vi "Continuous B sweep.vi"(6 "Mode":T2, 7 "Rate (T/min)":dbl=0.0125 min=0.0 max=0.2, 8 "error in (no error)":errorcluster, 9 "Simulate/Run":enum16{"simulate mode", "run mode"}(ring), 10 "Min (start)":dbl=1.0 min=-8.0 max=8.0, 11 "Max (end)":dbl=-1.0 min=-8.0 max=8.0) -> (0 "error out":errorcluster)   [LabVIEW 2019, in "Sweep Control.lvclass"]
uses:
  Sweep Control.lvclass
  Typedefs/Enum - Experiments.ctl
  Typedefs/Continuous B Sweep JSON--Cluster.ctl
  <userlib>/LevyLab/Transport/Transport/Transport.lvclass
  <userlib>/LevyLab/Transport/Control Experiment/Control Experiment.lvclass
  <userlib>/LevyLab/Instrument Framework/Instrument Types/Cryostat/Instrument.Cryostat.lvclass
  <userlib>/LevyLab/Transport/Control Experiment/Typedefs/Instrument Classes--cluster.ctl
  <userlib>/LevyLab/Transport/Control Experiment/Typedefs/Wiring Description--cluster.ctl
  <userlib>/LevyLab/Transport/Control Experiment/Typedefs/Experiment Description--cluster.ctl
  <userlib>/LevyLab/Instrument Framework/Instrument Types/VSource/Instrument.VSource.lvclass
  <userlib>/LevyLab/Instrument Framework/Instrument Types/VNA/Instrument.VNA.lvclass
  <userlib>/LevyLab/Instrument Framework/Instrument Types/Strain/Instrument.Strain.lvclass
  <userlib>/LevyLab/Instrument Framework/Instrument Types/CBridge/Instrument.CBridge.lvclass
  <userlib>/LevyLab/Lockin-Multichannel/Instrument.DAQ/Typedefs/Sweep.Pattern--Enum.ctl
  <userlib>/LevyLab/Lockin-Multichannel/Instrument.DAQ/Instrument.DAQ.lvclass
  <userlib>/LevyLab/Lockin-Multichannel/Instrument.DAQ/Typedefs/Sweep.Configuration--Cluster.ctl
  <userlib>/LevyLab/Instrument Framework/Instrument Types/Delay Line/Instrument.DelayLine.lvclass
  <userlib>/LevyLab/Lockin-Multichannel/Instrument.DAQ/Typedefs/REF.Channel--Cluster--Array.ctl
  <userlib>/LevyLab/Lockin-Multichannel/Instrument.DAQ/Typedefs/AO.Channel--Cluster--Array.ctl
  65c9b652-50f2-4ab4-8260-00ea008a43cc.vi
  <userlib>/LevyLab/Transport/Control Experiment/Typedefs/Instruments--cluster.ctl
  <userlib>/LevyLab/Krohn Hite 7008/KH7008/typedefs/Filter--Enum.ctl
  <userlib>/LevyLab/Krohn Hite 7008/KH7008/KH7008.lvlib
  <userlib>/LevyLab/Krohn Hite 7008/KH7008/typedefs/couple--Enum.ctl
  <userlib>/LevyLab/Krohn Hite 7008/KH7008/typedefs/shunt--enum.ctl
  <userlib>/LevyLab/Krohn Hite 7008/KH7008/typedefs/Input--Enum.ctl
  <userlib>/LevyLab/Krohn Hite 7008/KH7008/typedefs/gain--enum.ctl
  <userlib>/LevyLab/Krohn Hite 7008/KH7008/typedefs/channel--numeric.ctl
  <userlib>/LevyLab/Krohn Hite 7008/KH7008/typedefs/channelProperties--Cluster.ctl
  <userlib>/LevyLab/Krohn Hite 7008/KH7008/typedefs/allChannelProperties--Array.ctl
  <userlib>/LevyLab/Lockin-Multichannel/Instrument.DAQ/Typedefs/Sweep.Channel--Cluster.ctl
  <userlib>/LevyLab/Lockin-Multichannel/Instrument.DAQ/Typedefs/Sweep.Channel--Cluster--Array.ctl
  <userlib>/LevyLab/Instrument Framework/Instrument Types/Lockin/Instrument.LockinAPI.lvclass
  <userlib>/LevyLab/Instrument Framework/Instrument Types/Amplifier/Instrument.Amplifier.lvclass
  <userlib>/LevyLab/Lockin-Multichannel/Instrument.DAQ/Typedefs/AO.Channel.Function--Enum.ctl
  <userlib>/LevyLab/Lockin-Multichannel/Instrument.DAQ/Typedefs/AO.Channel--Cluster.ctl
  <userlib>/LevyLab/Lockin-Multichannel/Instrument.DAQ/Typedefs/REF.Channel--Cluster.ctl
  <userlib>/LevyLab/Lockin-Multichannel/Instrument.Lockin/Instrument.Lockin.lvclass
  <userlib>/LevyLab/Krohn Hite 7008/Inst.Krohn-Hite-7008/Inst.Krohn-Hite-7008.lvclass
  <userlib>/LevyLab/Instrument Framework/Instrument Types/Cryostat/Typedefs/Magnet Axis--Enum.ctl
  <userlib>/LevyLab/Transport/Control Experiment/Typedefs/Instrument Types--enum.ctl
  <userlib>/LevyLab/Instrument Framework/Instrument Types/Cryostat/Typedefs/Magnet Mode--Enum.ctl
  <userlib>/LevyLab/Transport/Transport/Typedefs/Lockin_Sweep JSON--Cluster.ctl
panel:
  in  "Lockin_sweep Configuration":T1[](array[typedef]) {"sweepTables"."Table" format="%#_3p"; "sweepTables"."Ch" min=1 max=16; "sweepChannels"."Table" format="%#_1f"; "sweepChannels"."Channel" min=1 max=128; "sweepChannels"."Start" format="%#_6p"; "sweepChannels"."End" format="%#_6p"}
  out "Setpoint (T)":dbl=1.0
  in  "Experiment Folder":string="49-LockinFieldSweep"
  in  "Experiment subVI":T3
  in  "Experiment Description":string="Lockin measurements at different X and Y gate values\n\n- lockin channel 17,18,19,20: leads 3,8,15,27 (x,y,-x,-y gates)\ngate combinations:\nx2,y2,x1,y1\n0,0,0,0\n17.5,0,-17.5,0\n-17.5,0,17.5,0\n0,17.5,0,-17.5\n0,-17.5,0,17.5\n17.5,0,17.5,0\n0,17.5,0,17.5\n\n-Vbg = lead 26: 0V\n-T: 20mK\n-B=1T to -1T @0.0125T/min and vice versa\n\n400nm periodicity hash\n\nLockin channel 2,1: leads 5,4 , current mode, SR: 5kOhm, Gain:1000x\nLockin channel 2: lead 5: Vac:1mV, Vdc:0V, freq: 13Hz\nLockin channel 3,4: leads 6,7 , voltage mode SR: open, Gain:1000x\n\nsolid rectangle\n    \nLockin channel 5,8: leads 9,13 , current mode, SR: 5kOhm, Gain:1000x\nLockin channel 5: lead 9: Vac:1mV, Vdc:0V, freq: 13Hz\nLockin channel 6,7: leads 11,12 , voltage mode SR: open, Gain:1000x\n\n\n200nm periodicity hash\n\nLockin channel 12,11: leads 21,20 , current mode, SR: 5kOhm, Gain:1000x\nLockin channel 12: lead 21: Vac:1mV, Vdc:0V, freq: 13Hz\nLockin channel 9,10: leads 16,17 , voltage mode SR: open, Gain:1000x\n\nAdditional lockin settings:\nLine filter on\nDecimation Factor: 10\nFs: 65000\n#s: 5000"
  out "time (minutes)":dbl=40.0
  out "ETA":timestamp=timestamp(3698546516.7356124 s since 1904-01-01) caption="Timestamp" format="%<%m/%d/%Y %I:%M:%S %p>T"
  out "time (hours)":dbl=2.0
  out "Step #":i32=1
  in  "Function":enum16{"Ramp", "Triangle", "Sine"}(ring)
  in  "Phase":dbl
  in  "Cycles (1,2,...)":i32=1 min=1 step=1
  in  "step size":dbl=2.0 format="%.4f"
  out "B Field Graph":cluster{i32[], dbl[]}[](graph)=[{[0, 1], [-1.0, 1.0]}, {[1], [1.0]}]
  in  "stop":bool
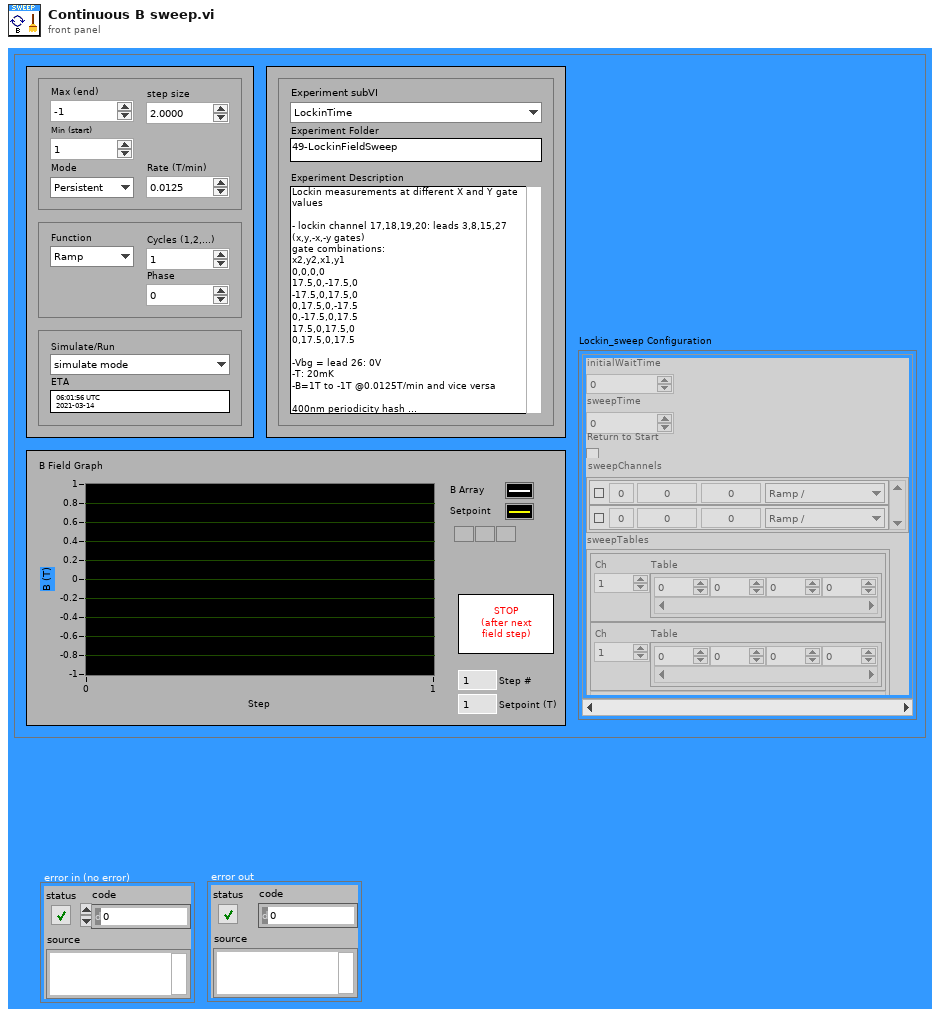
[diagram p1: front panel]
types:
  T1 = typedef "Transport.lvclass/Lockin_Sweep JSON--Cluster.ctl" = cluster{"initialWaitTime":dbl, "sweepTime":dbl, "Return to Start":bool, "sweepChannels":cluster{"Enable?":bool, "Channel":u16, "Start":dbl, "End":dbl, "Pattern":enum16{"Ramp /", "Ramp /\\", "Smooth Ramp _/", "Smooth Ramp _/\\_", "Table"}, "Table":dbl[]}[], "sweepTables":cluster{"Ch":i32, "Table":dbl[]}[]}
  T2 = typedef "Instrument.Cryostat.lvclass/Magnet Mode--Enum.ctl" = enum16{"Persistent", "Driven"}
  T3 = typedef "Sweep Control.lvclass/Enum - Experiments.ctl" = enum16{"LockinTime", "LockinSweep", "LockinDelayLine"}
  T4 = typedef "Instrument.Lockin.lvlib/Instrument.DAQ.lvclass/Sweep.Configuration--Cluster.ctl" = cluster{"sweepTime":dbl, "initialWaitTime":dbl, "returnToStart":bool, "sweepChannels":T5}
  T5 = typedef "Instrument.Lockin.lvlib/Instrument.DAQ.lvclass/Sweep.Channel--Cluster--Array.ctl" = T6[]
  T6 = typedef "Instrument.Lockin.lvlib/Instrument.DAQ.lvclass/Sweep.Channel--Cluster.ctl" = cluster{"Enable?":bool, "Channel":u16, "Start":dbl, "End":dbl, "Pattern":T7, "Table":dbl[]}
  T7 = typedef "Instrument.Lockin.lvlib/Instrument.DAQ.lvclass/Sweep.Pattern--Enum.ctl" = enum16{"Ramp /", "Ramp /\\", "Smooth Ramp _/", "Smooth Ramp _/\\_", "Table"}
  T8 = cluster{"Sweep Time (s)":dbl, "Initial Wait (s)":dbl, "Return to Start":bool, "Channels":T4[]}
  T9 = enum32{"Invalid", "Standard", "Closed", "Hidden", "Minimized", "Maximized"}
  T10 = enum32{"invalid app kind", "Development System", "Run Time System", "Student Edition", "Embedded LabVIEW", "Evaluation", "Custom"}
  T11 = typedef "Instrument.Cryostat.lvclass/Magnet Axis--Enum.ctl" = enum16{"X", "Y", "Z"}
  T12 = typedef "Sweep Control.lvclass/Continuous B Sweep JSON--Cluster.ctl" = cluster{"Continuous B Sweep":cluster{"Experiment":T3, "B field values":dbl[]}, "Experiment Description":T13, "Wiring Configuration":T16, "Lockin":cluster{"AOconfig":T17, "REFconfig":T20}, "Krohn Hite":cluster{"Channel Setting":T22}}
  T13 = typedef "Control Experiment.lvclass/Experiment Description--cluster.ctl" = cluster{"User":string, "Device":string, "Device Path":path, "Device Description":string, "Experiment Path":path, "Experiment Description":string, "Instrument":string, "Instruments":T14[], "Sweep":cluster{"key":string, "value":variant}[]}
  T14 = typedef "Control Experiment.lvclass/Instruments--cluster.ctl" = cluster{"class path":path, "Address":string, "Type":T15}
  T15 = typedef "Control Experiment.lvclass/Instrument Types--enum.ctl" = enum16{"DAQ", "Amplifier", "Temperature", "Magnet", "Rotator", "Level", "Capacitance", "Delay Line", "Strain Cell", "VNA", "Source"}
  T16 = typedef "Control Experiment.lvclass/Wiring Description--cluster.ctl" = cluster{"Lockin Ch":i32[], "KH":cluster{"Electrodes":string[], "Labels":string[]}, "not KH":cluster{"Electrodes":string[], "Labels":string[]}}
  T17 = typedef "Instrument.Lockin.lvlib/Instrument.DAQ.lvclass/AO.Channel--Cluster--Array.ctl" = T18[]
  T18 = typedef "Instrument.Lockin.lvlib/Instrument.DAQ.lvclass/AO.Channel--Cluster.ctl" = cluster{"Enable?":bool, "Channel":i32, "Amplitude":dbl, "Offset":dbl, "Frequency":dbl, "Phase":dbl, "Function":T19, "Sweeping?":bool, "Limit AC":bool, "Limit DC?":bool, "Duty Cycle":bool}
  T19 = typedef "Instrument.Lockin.lvlib/Instrument.DAQ.lvclass/AO.Channel.Function--Enum.ctl" = enum16{"sine", "square", "triangle", "saw"}
  T20 = typedef "Instrument.Lockin.lvlib/Instrument.DAQ.lvclass/REF.Channel--Cluster--Array.ctl" = T21[]
  T21 = typedef "Instrument.Lockin.lvlib/Instrument.DAQ.lvclass/REF.Channel--Cluster.ctl" = cluster{"Enable?":bool, "Channel":i32, "Frequency":dbl, "Phase":dbl, "TC":dbl, "Roll-Off":i32}
  T22 = typedef "KH7008.lvlib/allChannelProperties--Array.ctl" = T23[]
  T23 = typedef "KH7008.lvlib/channelProperties--Cluster.ctl" = cluster{"channel":T24, "gain":T25, "input":T26, "shunt":T27, "couple":T28, "filter":T29}
  T24 = typedef "KH7008.lvlib/channel--numeric.ctl" = u16
  T25 = typedef "KH7008.lvlib/gain--enum.ctl" = enum16{"1", "10", "100", "1000"}
  T26 = typedef "KH7008.lvlib/Input--Enum.ctl" = enum16{"OFF", "SE+", "SE-", "DIFF"}
  T27 = typedef "KH7008.lvlib/shunt--enum.ctl" = enum16{"Open", "50", "500", "5k", "50k", "10M"}
  T28 = typedef "KH7008.lvlib/couple--Enum.ctl" = enum16{"AC", "DC"}
  T29 = typedef "KH7008.lvlib/Filter--Enum.ctl" = enum16{"OFF", "ON"}
  T30 = typedef "Control Experiment.lvclass/Instrument Classes--cluster.ctl" = cluster{"DAQ":refnum<class "Instrument.LockinAPI.lvclass">, "Amplifier":refnum<class "Instrument.Amplifier.lvclass">, "Temperature":refnum<class "Instrument.Cryostat.lvclass">, "Magnet":refnum<class "Instrument.Cryostat.lvclass">, "Rotator":refnum<class "Instrument.Cryostat.lvclass">, "Level":refnum<class "Instrument.Cryostat.lvclass">, "Capacitance":refnum<class "Instrument.CBridge.lvclass">, "Delay Line":refnum<class "Instrument.DelayLine.lvclass">, "Strain Cell":refnum<class "Instrument.Strain.lvclass">, "VNA":refnum<class "Instrument.VNA.lvclass">, "Source":refnum<class "Instrument.VSource.lvclass">}
  T31 = cluster{"Core":cluster{"Current VI Reference":refnum<vi>, "Close Panel on Exit?":bool}, "SweepControl":refnum<class "Sweep Control.lvclass">, "ContinuousB_JSON":T12, "B field values":dbl[], "Sweep rate (T/min)":dbl, "Transport":refnum<class "Transport.lvclass">, "Instruments":T30}
  T32 = cluster{"Current VI Reference":refnum<vi>, "Close Panel on Exit?":bool}
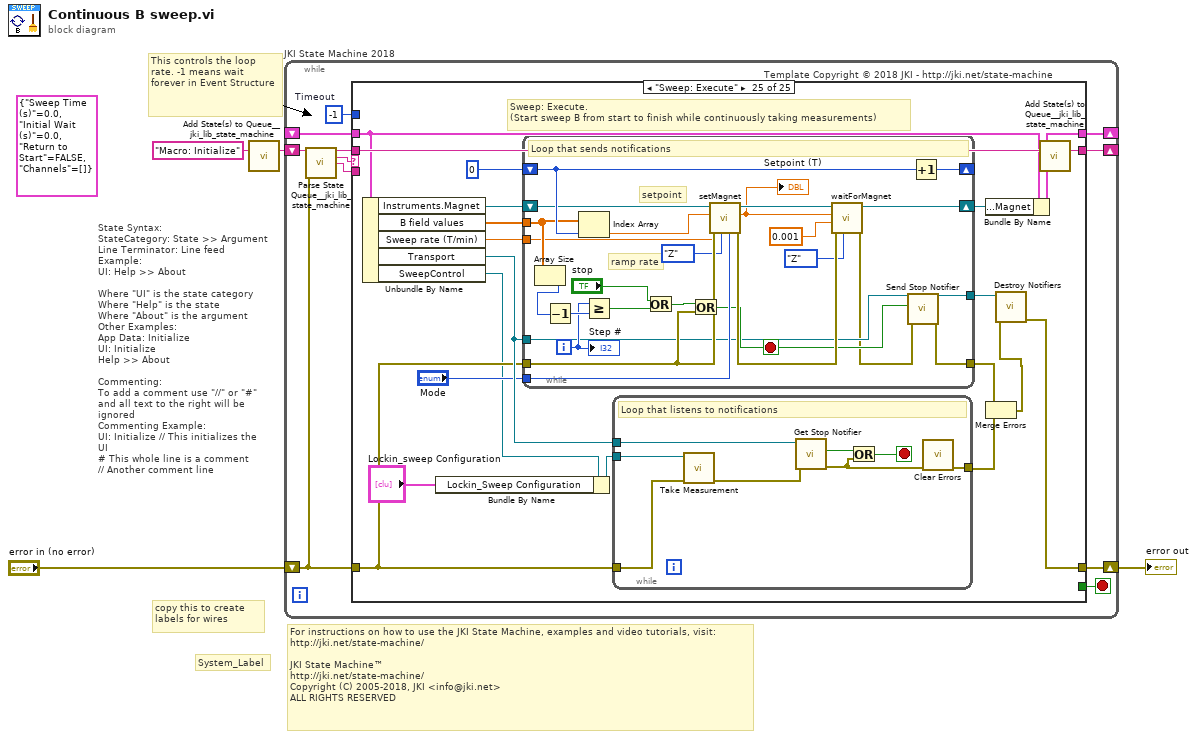
[diagram p0: block diagram]
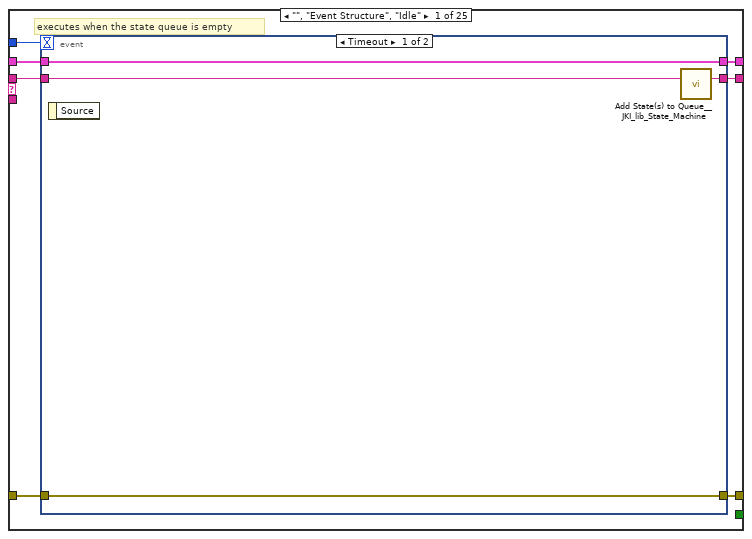
[diagram p2: hidden frame]
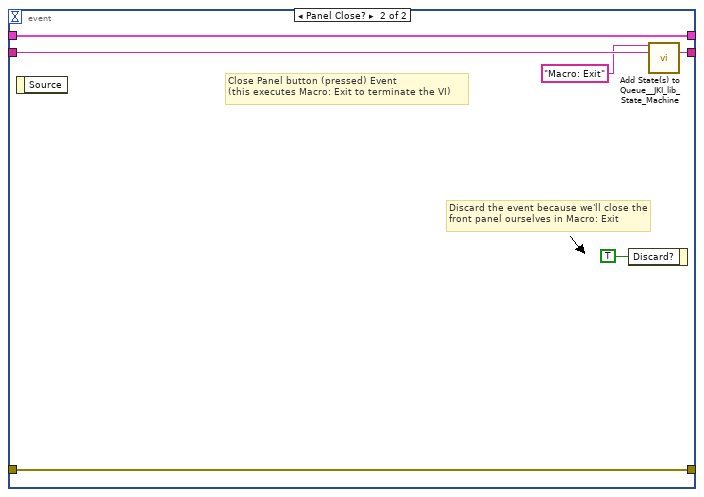
[diagram p3: hidden frame]
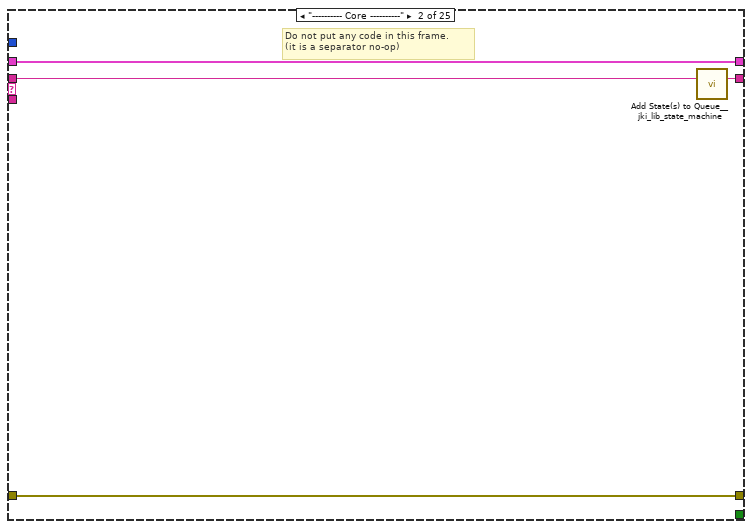
[diagram p4: hidden frame]
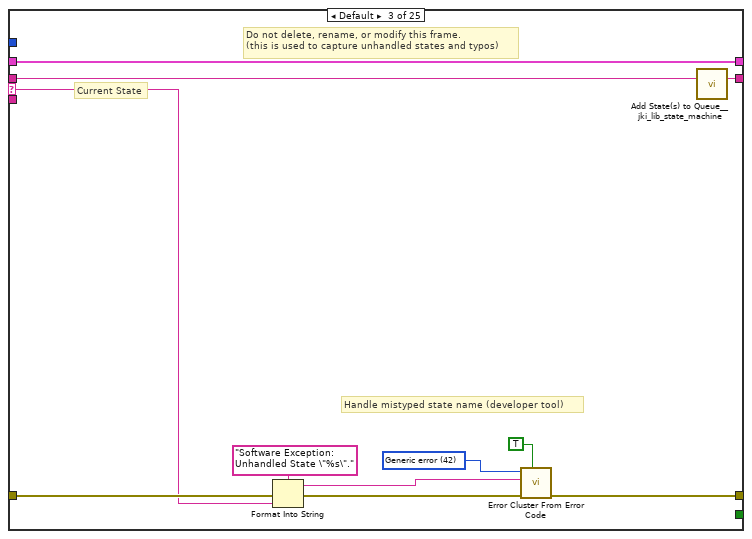
[diagram p5: hidden frame]
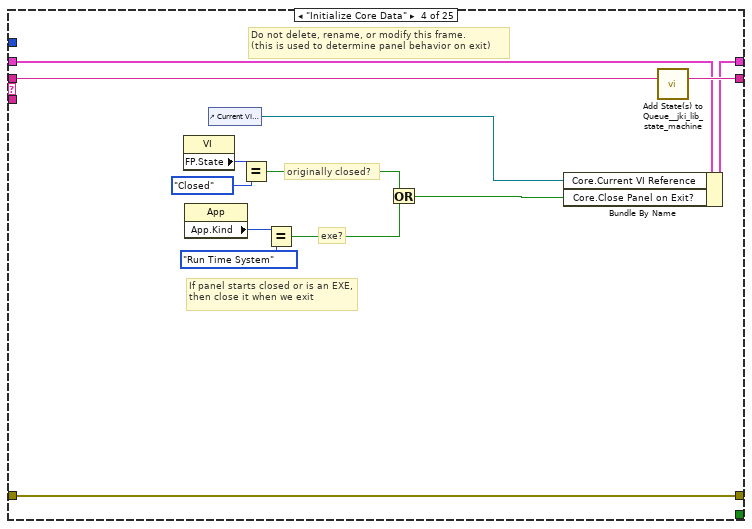
[diagram p6: hidden frame]
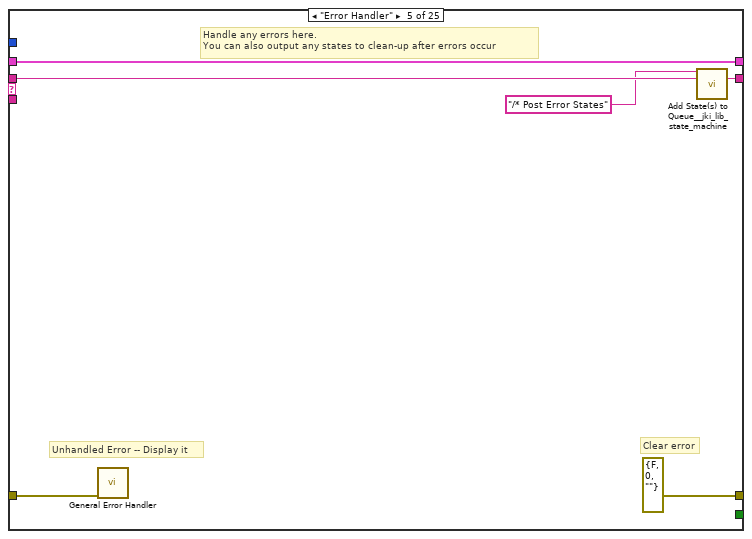
[diagram p7: hidden frame]
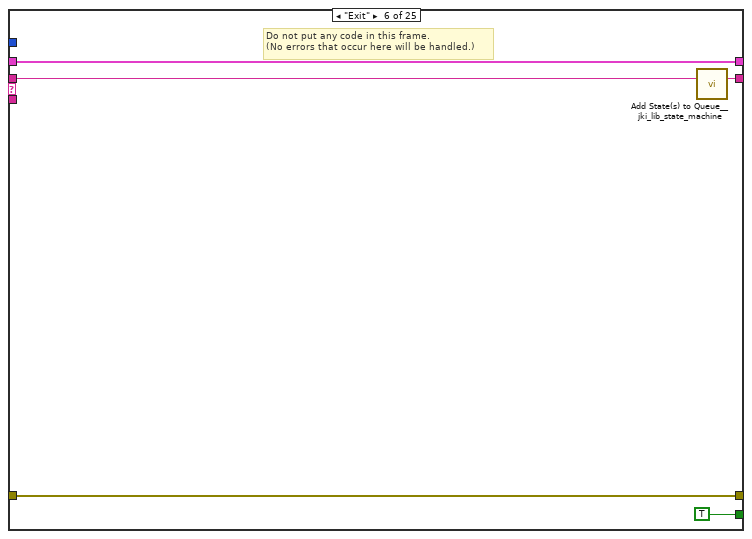
[diagram p8: hidden frame]
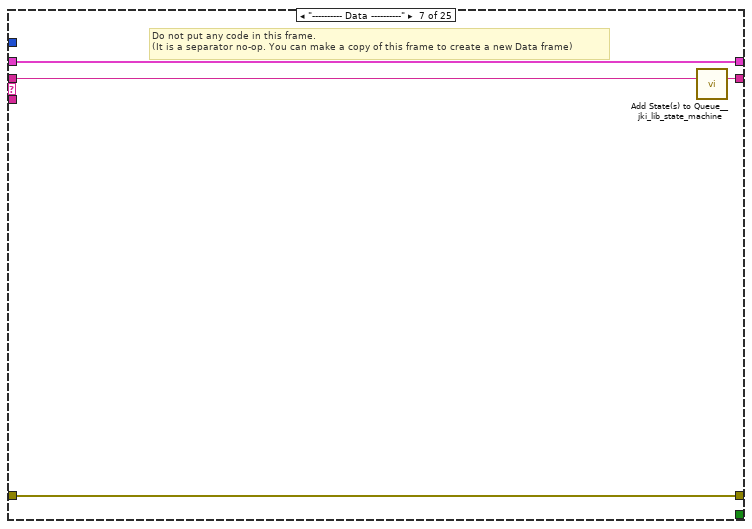
[diagram p9: hidden frame]
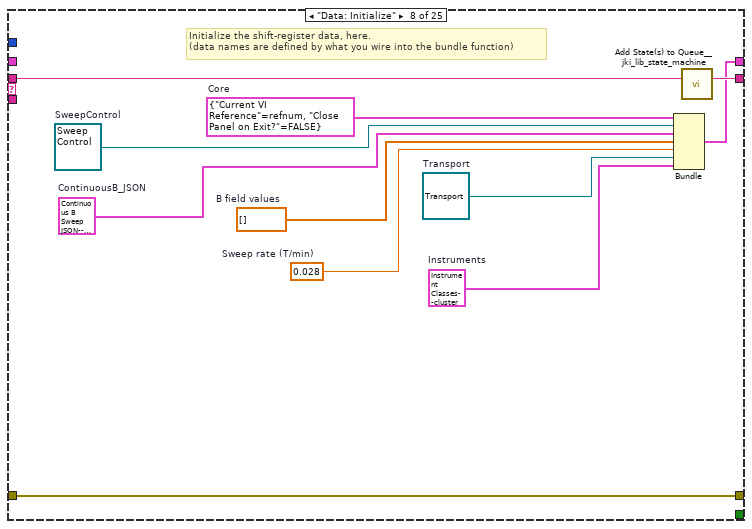
[diagram p10: hidden frame]
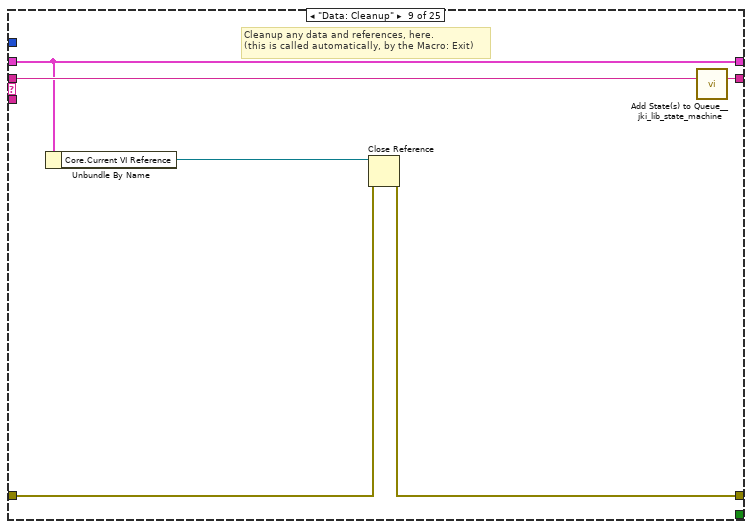
[diagram p11: hidden frame]
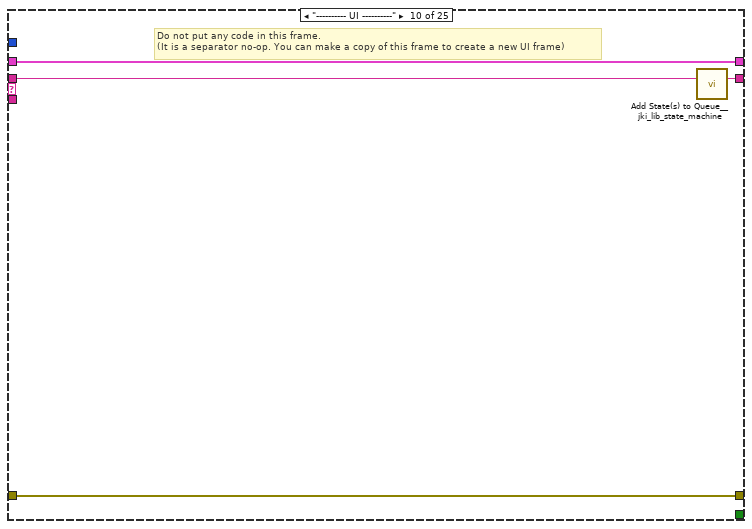
[diagram p12: hidden frame]
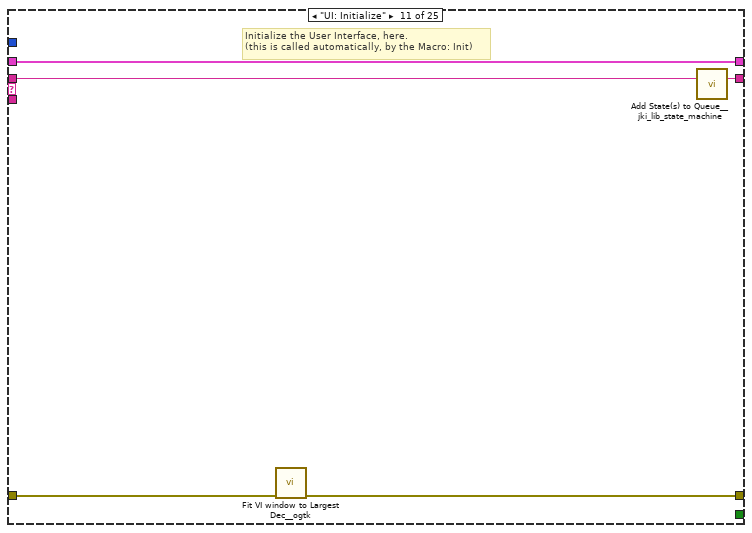
[diagram p13: hidden frame]
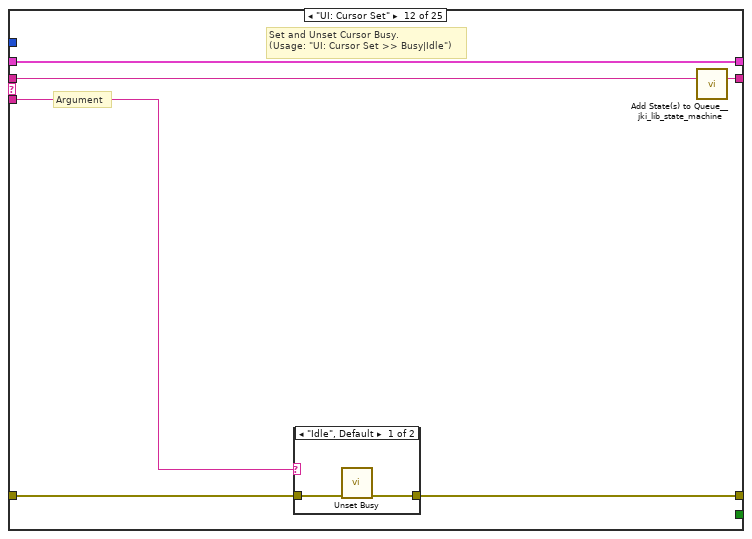
[diagram p14: hidden frame]
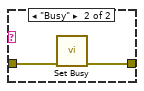
[diagram p15: hidden frame]
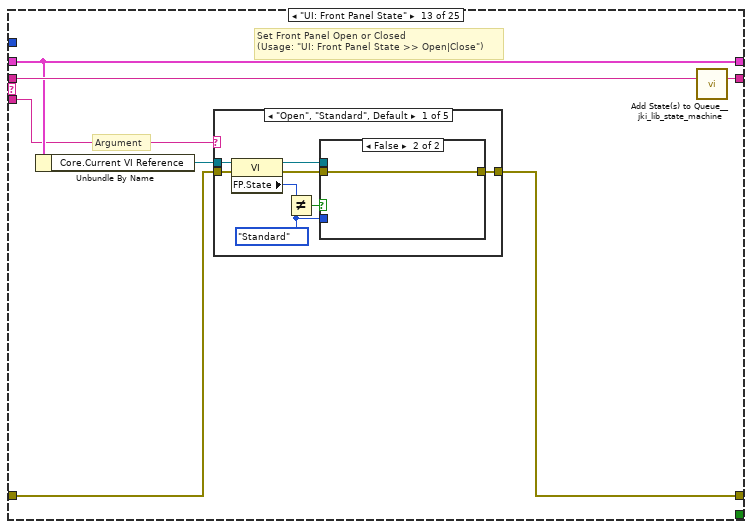
[diagram p16: hidden frame]
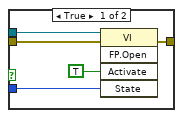
[diagram p17: hidden frame]
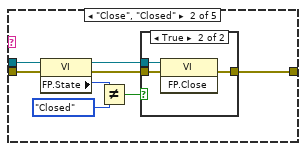
[diagram p18: hidden frame]
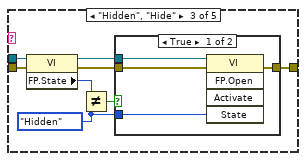
[diagram p20: hidden frame]
diagram:
  (unwired) T8 {"Sweep Time (s)"=0.0, "Initial Wait (s)"=0.0, "Return to Start"=FALSE, "Channels"=[]} ("Sweep")
  # "For instructions on how to use the JKI State Machine, examples and video tutorials, visit:\nhttp://jki.net/state-machine/\n\nJKI State Machine™\nhttp://jki.net/state-machine/\nCopyright (C) 2005-2018, JKI <info@jki.net>\nALL RIGHTS RESERVED"
  # "State Syntax:\nStateCategory: State >> Argument\nLine Terminator: Line feed\nExample:\nUI: Help >> About\n\nWhere \"UI\" is the state category\nWhere \"Help\" is the state\nWhere \"About\" is the argument\nOther Examples:\nApp Data: Initialize\nUI: Initialize\nHelp >> About\n\nCommenting:\nTo add a comment use \"//\" or \"#\" and all text to the right will be ignored\nCommenting Example:\nUI: Initialize // This initializes the UI\n# This whole line is a comment\n// Another comment line"
  # "copy this to create labels for wires"
  # "This controls the loop rate. -1 means wait forever in Event Structure"
  # "System_Label"
  n1 = call <vilib>:"Add State(s) to Queue__jki_lib_state_machine.vi"("State(s) in (\"\")"="Macro: Initialize") -> ("States Out"=w4:string)  [unwired: 14 in]
  n2 = while "JKI State Machine 2018" {
    shift-right: [w8] -> _
    shift-left: _ -> [w7]
    shift-right: [w11] -> w1
    shift-left: "error in (no error)" -> [w5]
    shift-right: [w10] -> _
    shift-left: w4 -> [w12]
    stop <- w9 stop-if-true
    w6 = -1  # Timeout
    # "Template Copyright © 2018 JKI - http://jki.net/state-machine"
    n3 = call <vilib>:"Parse State Queue__jki_lib_state_machine.vi"("State Queue"=w12, "Error In (no error)"=w5) -> ("Remaining States"=w14:string, "Current State"=w15:string, "Arguments"=w13:string)  [unwired: 11 in]
    n4 = case shown="\"Sweep: Execute\"" w15 {
      selector: w15 -> [_ _ w37 _ _ _ _ _ _ _ _ _ _ _ _ _ _ _ _ _ _ _ _ _ _]
      tunnel: w14 -> [w22 w36 w41 w60 w66 w71 w75 w86 w92 w96 w101 w107 w118 w187 w192 w201 w213 w217 w236 w262 w275 w308 w336 w353 w392]
      tunnel: w13 -> [_ _ _ _ _ _ _ _ _ _ _ w102 w112 _ _ _ _ _ _ _ _ _ _ _ _]
      tunnel: w7 -> [w20 w33 w39 w53 w63 w69 w72 _ w87 w93 w99 w105 w114 w184 w189 w198 w210 w214 w226 w248 w272 w300 w334 w340 w380]
      tunnel: [w19 w34 w43 w57 errorcluster {"status"=FALSE, "code"=0, "source"=""} ("error out") w68 w73 w83 w88 w94 w97 w103 w115 w185 w190 w199 w211 w215 w224 w239 w263 w294 w318 w351 w373] -> w11
      tunnel: w5 -> [w18 w34 w42 w57 w62 w68 w73 w83 w89 w94 w98 w104 w116 w185 w190 w199 w211 w215 w224 w252 w266 w283 w323 w351 w386]
      tunnel: [w21 w35 w40 w59 w65 w70 w74 w85 w91 w95 w100 w106 w117 w186 w191 w200 w212 w216 w235 w261 w274 w307 w335 w352 w391] -> w10
      tunnel: [_ _ _ _ _ TRUE _ _ _ _ _ _ _ _ _ _ _ _ _ _ _ _ _ _ _] -> w9
      tunnel: [w17 w33 w39 w58 w63 w69 w72 w84 w87 w93 w99 w105 w114 w184 w189 w198 w210 w214 w234 w247 w273 w299 w333 w340 w379] -> w8
      tunnel: w6 -> [w16 _ _ _ _ _ _ _ _ _ _ _ _ _ _ _ _ _ _ _ _ _ _ _ _]
      frame "", "Event Structure", "Idle" {
        # "executes when the state queue is empty"
        n5 = event shown="[0] Timeout" {
          selector: _ -> [_ _]
          dyn-events: _ -> [_ _]
          timeout: w16 -> [_ _]
          tunnel: w22 -> [w26 w32]
          tunnel: [w25 w31] -> w21
          tunnel: w20 -> [w23 w29]
          tunnel: [w24 w30] -> w19
          tunnel: w18 -> [w24 w30]
          tunnel: [w23 w29] -> w17
          event Timeout {
            n6 = event-data() -> ()  [unwired: 1 in, 1 out]
            n7 = call <vilib>:"Add State(s) to Queue__JKI_lib_State_Machine.vi"("State(s) in (\"\")"=w26) -> ("States Out"=w25:string)  [unwired: 14 in]
          }
          event Panel Close? {
            # "Discard the event because we'll close the front panel ourselves in Macro: Exit"
            # "Close Panel button (pressed) Event\n(this executes Macro: Exit to terminate the VI)"
            n8 = event-data() -> ()  [unwired: 1 in, 1 out]
            n9 = event-data("Discard?"=TRUE) -> ()  [unwired: 1 in, 1 out]
            n10 = call <vilib>:"Add State(s) to Queue__JKI_lib_State_Machine.vi"("State(s) in Front (\"\")"="Macro: Exit", "State(s) in (\"\")"=w32) -> ("States Out"=w31:string)  [unwired: 13 in]
          }
        }
      }
      frame "---------- Core ----------" {
        # "Do not put any code in this frame.\n(it is a separator no-op)"
        n11 = call <vilib>:"Add State(s) to Queue__jki_lib_state_machine.vi"("State(s) in (\"\")"=w36) -> ("States Out"=w35:string)  [unwired: 14 in]
      }
      frame Default {
        w46 = 42 items=["No error", "Argument error", "Memory is full", "Out of zone", "End of file", "File already open", "Generic file I/O error", "File not found", "File permission error", "Disk is full", "Duplicate path", "Too many files open", "System feature not enabled", "Resource file not found", "Cannot add resource", "Resource not found", "Image not found", "Image memory error", "Pen does not exist", "Config type invalid", "Config token not found", "Config parse error", "Config memory error", "Bad external code format", "Bad external code offset", "External code not present", "Null window", "Destroy window error", "Null menu", "Print aborted", "Bad print record", "Print driver error", "Windows error during printing", "Memory error during printing", "Print dialog error", "Generic print error", "Invalid device refnum", "Device not found", "Device parameter error", "Device unit error", "Cannot open device", "Device call aborted", "Generic error", "Cancelled by user", "Object ID too low", "Object ID too high", "Object not in heap", "Unknown heap", "Unknown object (invalid DefProc)", "Unknown object (DefProc not in table)", "Message out of range", "Invalid (null) method", "Unknown message", "Manager call not supported", "Bad address", "Network operation in progress", "Network operation timed out", "Connection is busy", "Network attribute not supported", "Network error", "Address in use", "System out of memory", "Connection aborted", "Connection refused", "Not connected", "Already connected", "Connection closed", "Initialization error (interapplication manager)", "Bad occurrence", "Wait on unbound occurrence handler", "Occurrence queue overflow", "Datalog type conflict", "Unused", "Unrecognized type (interapplication manager)", "Memory corrupt", "Failed to make temporary DLL", "Old CIN version", "Drag socket not found", "Failed to load drop-object", "Failed to register OLE object", "Failed to release OLE object", "Format specifier type mismatch", "Unknown format specifier", "Too few format specifiers", "Too many format specifiers", "Scan failed", "Newer CIN version", "Error converting to variant", "Runtime menu error", "Password tampered", "Variant attribute not found", "Incompatible variant data type", "Event data is not available", "Event Store is not present", "Occurrence is not found", "Event Queue is not created", "Event info is not available", "Refnum passed is NULL", "Error retrieving Class GUID", "Error retrieving CoClass GUID", "Error retrieving TypeLib GUID.", "Bad built application magic bytes.", "Specific driver is different from the specific driver associated with the Logical Name.", "There is no session opened to the class driver.", "Max Error", "MAX - Error with config objects", "MAX - Error loading configuration", "MAX - Group not supported"]
        # "Current State"
        # "Do not delete, rename, or modify this frame.\n(this is used to capture unhandled states and typos)"
        # "Handle mistyped state name (developer tool)"
        n12 = Format Into String(format string="Software Exception: Unhandled State \"%s\"." ("message"), error in=w42, w37) -> (resulting string=w45:string, error out=w44:errorcluster)  [unwired: 1 in]
        n13 = call <vilib>:"Error Cluster From Error Code.vi"("show call chain? (False)"=TRUE, "error in (no error)"=w44, "error message (\"\")"=w45, "error code (0)"=w46) -> ("error out"=w43:errorcluster)  [unwired: 5 in]
        n14 = call <vilib>:"Add State(s) to Queue__jki_lib_state_machine.vi"("State(s) in (\"\")"=w41) -> ("States Out"=w40:string)  [unwired: 14 in]
      }
      frame "Initialize Core Data" {
        # "Do not delete, rename, or modify this frame.\n(this is used to determine panel behavior on exit)"
        # "originally closed?"
        # "exe?"
        # "If panel starts closed or is an EXE, then close it when we exit"
        n15 = property class="VI"() -> ("FP.State"=w50:T9)  [unwired: 2 in, 2 out]
        n16 = property class="App"() -> ("App.Kind"=w56:T10)  [unwired: 2 in, 2 out]
        n17 = control-ref of="Current VI Reference"() -> (w51:refnum<vi>)
        n18 = Equal?(x=w50, y=T9."Closed" ("Front Panel Window:State")) -> (x = y?=w48:bool)
        n19 = Equal?(x=w56, y=T10."Run Time System" ("Application:Kind")) -> (x = y?=w54:bool)
        n20 = Or(x=w48, y=w54) -> (x .or. y?=w52:bool)
        n21 = Bundle By Name(cluster=w53, "Core.Current VI Reference"=w51, "Core.Close Panel on Exit?"=w52) -> (w58:T31)
        n22 = call <vilib>:"Add State(s) to Queue__jki_lib_state_machine.vi"("State(s) in (\"\")"=w60) -> ("States Out"=w59:string)  [unwired: 14 in]
      }
      frame "Error Handler" {
        # "Unhandled Error -- Display it"
        # "Handle any errors here.\nYou can also output any states to clean-up after errors occur"
        # "Clear error"
        n23 = call <vilib>:"General Error Handler.vi"("error in (no error)"=w62) -> ()  [unwired: 10 in, 5 out]
        n24 = call <vilib>:"Add State(s) to Queue__jki_lib_state_machine.vi"("State(s) in Front (\"\")"="/* Post Error States", "State(s) in (\"\")"=w66) -> ("States Out"=w65:string)  [unwired: 13 in]
      }
      frame "Exit" {
        # "Do not put any code in this frame.\n(No errors that occur here will be handled.)"
        n25 = call <vilib>:"Add State(s) to Queue__jki_lib_state_machine.vi"("State(s) in (\"\")"=w71) -> ("States Out"=w70:string)  [unwired: 14 in]
      }
      frame "---------- Data ----------" {
        # "Do not put any code in this frame.\n(It is a separator no-op. You can make a copy of this frame to create a new Data frame)"
        n26 = call <vilib>:"Add State(s) to Queue__jki_lib_state_machine.vi"("State(s) in (\"\")"=w75) -> ("States Out"=w74:string)  [unwired: 14 in]
      }
      frame "Data: Initialize" {
        w77 = T12 {"Continuous B Sweep"={"Experiment"=enum."LockinDelayLine", "B field values"=[]}, "Experiment Description"={"User"="", "Device"="", "Device Path"=path "", "Device Description"="", "Experiment Path"=path "", "Experiment Description"="", "Instrument"="", "Instruments"=[], "Sweep"=[]}, "Wiring Configuration"={"Lockin Ch"=[], "KH"={"Electrodes"=[], "Labels"=[]}, "not KH"={"Electrodes"=[], "Labels"=[]}}, "Lockin"={"AOconfig"=[], "REFconfig"=[]}, "Krohn Hite"={"Channel Setting"=[]}}  # ContinuousB_JSON
        w78 = T30 {"DAQ"=refnum, "Amplifier"=refnum, "Temperature"=refnum, "Magnet"=refnum, "Rotator"=refnum, "Level"=refnum, "Capacitance"=refnum, "Delay Line"=refnum, "Strain Cell"=refnum, "VNA"=refnum, "Source"=refnum}  # Instruments
        w76 = refnum<class "Transport.lvclass"> refnum  # Transport
        w79 = refnum<class "Sweep Control.lvclass"> refnum  # SweepControl
        w80 = 0.028  # Sweep rate (T/min)
        w81 = dbl[] []  # B field values
        w82 = T32 {"Current VI Reference"=refnum, "Close Panel on Exit?"=FALSE}  # Core
        # "Initialize the shift-register data, here.\n(data names are defined by what you wire into the bundle function)"
        n27 = Bundle("Core"=w82, "SweepControl"=w79, "ContinuousB_JSON"=w77, "B field values"=w81, "Sweep rate (T/min)"=w80, "Transport"=w76, "Instruments"=w78) -> (w84:T31)  [unwired: 1 in]
        n28 = call <vilib>:"Add State(s) to Queue__jki_lib_state_machine.vi"("State(s) in (\"\")"=w86) -> ("States Out"=w85:string)  [unwired: 14 in]
      }
      frame "Data: Cleanup" {
        # "Cleanup any data and references, here.\n(this is called automatically, by the Macro: Exit)"
        n29 = Unbundle By Name(w87) -> ("Core.Current VI Reference"=w90:refnum<vi>)
        n30 = Close Reference(reference=w90, error in (no error)=w89) -> (error out=w88:errorcluster)
        n31 = call <vilib>:"Add State(s) to Queue__jki_lib_state_machine.vi"("State(s) in (\"\")"=w92) -> ("States Out"=w91:string)  [unwired: 14 in]
      }
      frame "---------- UI ----------" {
        # "Do not put any code in this frame.\n(It is a separator no-op. You can make a copy of this frame to create a new UI frame)"
        n32 = call <vilib>:"Add State(s) to Queue__jki_lib_state_machine.vi"("State(s) in (\"\")"=w96) -> ("States Out"=w95:string)  [unwired: 14 in]
      }
      frame "UI: Initialize" {
        # "Initialize the User Interface, here.\n(this is called automatically, by the Macro: Init)"
        n33 = call <userlib>:"Fit VI window to Largest Dec__ogtk.vi"("error in (no error)"=w98) -> ("error out"=w97:errorcluster)  [unwired: 5 in, 1 out]
        n34 = call <vilib>:"Add State(s) to Queue__jki_lib_state_machine.vi"("State(s) in (\"\")"=w101) -> ("States Out"=w100:string)  [unwired: 14 in]
      }
      frame "UI: Cursor Set" {
        # "Argument"
        # "Set and Unset Cursor Busy.\n(Usage: \"UI: Cursor Set >> Busy|Idle\")"
        n35 = case shown="\"Idle\", Default" w102 {
          tunnel: w104 -> [w109 w111]
          tunnel: [w108 w110] -> w103
          frame "Idle", Default {
            n36 = call <vilib>:"Unset Busy.vi"("error in (no error)"=w109) -> ("error out"=w108:errorcluster)  [unwired: 10 in]
          }
          frame "Busy" {
            n37 = call <vilib>:"Set Busy.vi"("error in (no error)"=w111) -> ("error out"=w110:errorcluster)  [unwired: 9 in, 1 out]
          }
        }
        n38 = call <vilib>:"Add State(s) to Queue__jki_lib_state_machine.vi"("State(s) in (\"\")"=w107) -> ("States Out"=w106:string)  [unwired: 14 in]
      }
      frame "UI: Front Panel State" {
        # "Argument"
        # "Set Front Panel Open or Closed\n(Usage: \"UI: Front Panel State >> Open|Close\")"
        n39 = Unbundle By Name(w114) -> ("Core.Current VI Reference"=w113:refnum<vi>)
        n40 = case shown="\"Open\", \"Standard\", Default" w112 {
          tunnel: w116 -> [w124 w139 w150 w163 w176]
          tunnel: [w126 w140 w152 w165 w178] -> w115
          tunnel: w113 -> [w125 w137 w151 w164 w177]
          frame "Open", "Standard", Default {
            w119 = T9."Standard" ("State")
            n41 = property class="VI"(reference=w125, error in=w124) -> (reference out=w122:refnum<vi>, error out=w123:errorcluster, "FP.State"=w121:T9)
            n42 = Not Equal?(x=w121, y=w119) -> (x != y?=w120:bool)
            n43 = case shown="False" w120 {
              tunnel: [w130 w132] -> w126
              tunnel: w123 -> [w129 w132]
              tunnel: w122 -> [w128 _]
              tunnel: w119 -> [w127 _]
              frame True {
                n44 = invoke class="VI" method="FP.Open"(reference=w128, error in=w129, "Activate"=TRUE, "State"=w127) -> (error out=w130:errorcluster)  [unwired: 1 in, 4 out]
              }
              frame False {
              }
            }
          }
          frame "Close", "Closed" {
            n45 = property class="VI"(reference=w137, error in=w139) -> (reference out=w136:refnum<vi>, error out=w138:errorcluster, "FP.State"=w134:T9)
            n46 = Not Equal?(x=w134, y=T9."Closed" ("Front Panel Window:State")) -> (x != y?=w133:bool)
            n47 = case shown="True" w133 {
              tunnel: [w141 w144] -> w140
              tunnel: w138 -> [w141 w143]
              tunnel: w136 -> [_ w142]
              frame False {
              }
              frame True {
                n48 = invoke class="VI" method="FP.Close"(reference=w142, error in=w143) -> (error out=w144:errorcluster)  [unwired: 1 in, 2 out]
              }
            }
          }
          frame "Hidden", "Hide" {
            w145 = T9."Hidden" ("State")
            n49 = property class="VI"(reference=w151, error in=w150) -> (reference out=w148:refnum<vi>, error out=w149:errorcluster, "FP.State"=w147:T9)
            n50 = Not Equal?(x=w147, y=w145) -> (x != y?=w146:bool)
            n51 = case shown="True" w146 {
              tunnel: [w156 w157] -> w152
              tunnel: w149 -> [w155 w157]
              tunnel: w148 -> [w154 _]
              tunnel: w145 -> [w153 _]
              frame True {
                n52 = invoke class="VI" method="FP.Open"(reference=w154, error in=w155, "State"=w153) -> (error out=w156:errorcluster)  [unwired: 2 in, 4 out]
              }
              frame False {
              }
            }
          }
          frame "Minimize", "Minimized" {
            w158 = T9."Minimized" ("State")
            n53 = property class="VI"(reference=w164, error in=w163) -> (reference out=w161:refnum<vi>, error out=w162:errorcluster, "FP.State"=w160:T9)
            n54 = Not Equal?(x=w160, y=w158) -> (x != y?=w159:bool)
            n55 = case shown="True" w159 {
              tunnel: [w169 w170] -> w165
              tunnel: w162 -> [w168 w170]
              tunnel: w161 -> [w167 _]
              tunnel: w158 -> [w166 _]
              frame True {
                n56 = invoke class="VI" method="FP.Open"(reference=w167, error in=w168, "State"=w166) -> (error out=w169:errorcluster)  [unwired: 2 in, 4 out]
              }
              frame False {
              }
            }
          }
          frame "Maximize", "Maximized" {
            w171 = T9."Maximized" ("State")
            n57 = property class="VI"(reference=w177, error in=w176) -> (reference out=w174:refnum<vi>, error out=w175:errorcluster, "FP.State"=w173:T9)
            n58 = Not Equal?(x=w173, y=w171) -> (x != y?=w172:bool)
            n59 = case shown="True" w172 {
              tunnel: [w182 w183] -> w178
              tunnel: w175 -> [w181 w183]
              tunnel: w174 -> [w180 _]
              tunnel: w171 -> [w179 _]
              frame True {
                n60 = invoke class="VI" method="FP.Open"(reference=w180, error in=w181, "State"=w179) -> (error out=w182:errorcluster)  [unwired: 2 in, 4 out]
              }
              frame False {
              }
            }
          }
        }
        n61 = call <vilib>:"Add State(s) to Queue__jki_lib_state_machine.vi"("State(s) in (\"\")"=w118) -> ("States Out"=w117:string)  [unwired: 14 in]
      }
      frame "---------- Macro ----------" {
        # "Do not put any code in this frame.\n(It is a separator no-op. You can make a copy of this frame to create a new Macro frame)"
        n62 = call <vilib>:"Add State(s) to Queue__jki_lib_state_machine.vi"("State(s) in (\"\")"=w187) -> ("States Out"=w186:string)  [unwired: 14 in]
      }
      frame "Macro: Initialize" {
        w188 = "Data: Initialize\nInitialize Core Data\nUI: Initialize\nUI: Front Panel State >> Open\nMacro: Sweep"  # Data: Initialize Initialize Core Data UI: Initialize UI: Front Panel State >> Open Macro: Sweep
        # "Initialization Macro\n(This is called once, when the VI starts)"
        n63 = call <vilib>:"Add State(s) to Queue__jki_lib_state_machine.vi"("State(s) in Front (\"\")"=w188, "State(s) in (\"\")"=w192) -> ("States Out"=w191:string)  [unwired: 13 in]
      }
      frame "Macro: Sweep" {
        # "Macro: Sweep.\n(Initialize Sweep, Execute or Simulate Sweep, Exit)"
        n64 = case shown="\"run mode\"" "Simulate/Run" {
          tunnel: ["Sweep: Simulate Sweep" "Sweep: Initialize Sweep Control\nSweep: Initialize Transport\nSweep: Prepare JSON\nSweep: Write JSON\nSweep: Execute"] -> w196
          frame "simulate mode", Default {
          }
          frame "run mode" {
          }
        }
        n65 = call <vilib>:"Add State(s) to Queue__jki_lib_state_machine.vi"("State(s) in Front (\"\")"="Sweep: Initialize", "State(s) in (\"\")"=w196, "State(s) at Back (\"\")"="Macro: Exit") -> ("States Out"=w195:string)  [unwired: 12 in]
        n66 = call <vilib>:"Add State(s) to Queue__jki_lib_state_machine.vi"("State(s) in Front (\"\")"=w195, "State(s) in (\"\")"=w201) -> ("States Out"=w200:string)  [unwired: 13 in]
      }
      frame "Macro: Exit" {
        # "Exit Macro\n(This is called once, when the VI exits)"
        n67 = Unbundle By Name(w210) -> ("Core.Close Panel on Exit?"=w209:bool)
        n68 = Select(t="UI: Front Panel State >> Close", s=w209, f="") -> (s? t:f=w206:string)
        n69 = call <vilib>:"Add State(s) to Queue__JKI_lib_State_Machine.vi"("State(s) in (\"\")"=w206, "State(s) at Back (\"\")"="Data: Cleanup\nExit") -> ("States Out"=w204:string)  [unwired: 13 in]
        n70 = call <vilib>:"Add State(s) to Queue__jki_lib_state_machine.vi"("State(s) in Front (\"\")"=w204, "State(s) in (\"\")"=w213) -> ("States Out"=w212:string)  [unwired: 13 in]
      }
      frame "---------- Sweep ----------" {
        # "Template Separator\n(You can make a copy of, or modify, this frame)"
        n71 = call <vilib>:"Add State(s) to Queue__jki_lib_state_machine.vi"("State(s) in (\"\")"=w217) -> ("States Out"=w216:string)  [unwired: 14 in]
      }
      frame "Sweep: Initialize" {
        # "Sweep: Initialize.\n(Initialize sweep waypoints)"
        n72 = call <userlib>:"Max_Min_conversion.vi"("Min"="Min (start)", "Max"="Max (end)") -> ("offset"=w229:dbl, "Amplitude"=w228:dbl)  [unwired: 8 in]
        n73 = call <userlib>:"Ramp.vi"("phase"="Phase", "function (ramp)"="Function", "cycles (1,2,...)"="Cycles (1,2,...)", "step size"="step size", "offset"=w229, "amplitude"=w228) -> ("Waveform Graph"=w222:dbl[])  [unwired: 3 in, 2 out]
        n74 = for {
          tunnel: w222 -> [w237] mode=indexing
          tunnel: [w238] -> w221 mode=indexing
          tunnel: [w237] -> w220 mode=indexing
          i -> [w238]
        }
        n75 = Bundle(w221, w220) -> (w219:cluster{i32[], dbl[]})  [unwired: 1 in]
        n76 = Build Array(w219) -> (→"B Field Graph":cluster{i32[], dbl[]}[])
        n77 = Bundle By Name(cluster=w226, "B field values"=w222, "Sweep rate (T/min)"="Rate (T/min)") -> (w234:T31)
        n78 = call <vilib>:"Add State(s) to Queue__jki_lib_state_machine.vi"("State(s) in (\"\")"=w236) -> ("States Out"=w235:string)  [unwired: 14 in]
      }
      frame "Sweep: Initialize Sweep Control" {
        # "Sweep: Initialize Sweep Control\n(Read Control Experiment.json, Sets Experiment Description and Folder)"
        n79 = Unbundle By Name(w248) -> ("SweepControl"=w253:refnum<class "Sweep Control.lvclass">)
        n80 = call <userlib>:"Control Experiment FGV.vi"("Function"=enum16{"read", "write"}."read", "error in (no error)"=w252) -> ("error out"=w249:errorcluster, "Control Experiment.lvclass out"=w258:refnum<class "Control Experiment.lvclass">)  [unwired: 6 in, 2 out]
        n81 = Bundle By Name(cluster=w253, "Experiment"="Experiment subVI") -> (w242:refnum<class "Sweep Control.lvclass">)
        n82 = call <userlib>:"Write Experiment Description.vi"("error in (no error)"=w249, "Experiment Description"="Experiment Description", "Control Experiment in"=w258) -> ("error out"=w250:errorcluster, "Control Experiment out"=w257:refnum<class "Control Experiment.lvclass">)  [unwired: 7 in]
        n83 = call <userlib>:"Write Experiment Folder.vi"("error in (no error)"=w250, "Experiment Folder"="Experiment Folder", "Control Experiment in"=w257) -> ("error out"=w251:errorcluster, "Control Experiment out"=w259:refnum<class "Control Experiment.lvclass">)  [unwired: 7 in]
        n84 = call <userlib>:"Read Instruments.vi"("error in (no error)"=w251, "Control Experiment in"=w259) -> ("error out"=w244:errorcluster, "Instruments"=w246:T30, "Control Experiment out"=w245:refnum<class "Control Experiment.lvclass">)  [unwired: 7 in]
        n85 = call <userlib>:"Write Dependencies.vi"("error in (no error)"=w244, "Control Experiment"=w245) -> ("error out"=w240:errorcluster, "Transport out"=w243:refnum<class "Transport.lvclass">)  [unwired: 8 in]
        n86 = call <userlib>:"Write Dependencies.vi"("error in (no error)"=w240, "Transport"=w243, "SweepControl in"=w242) -> ("error out"=w239:errorcluster, "SweepControl out"=w241:refnum<class "Sweep Control.lvclass">)  [unwired: 7 in]
        n87 = Bundle By Name(cluster=w248, "SweepControl"=w241, "Instruments"=w246) -> (w247:T31)
        n88 = call <vilib>:"Add State(s) to Queue__jki_lib_state_machine.vi"("State(s) in (\"\")"=w262) -> ("States Out"=w261:string)  [unwired: 14 in]
      }
      frame "Sweep: Initialize Transport" {
        # "Sweep: Initialize Transport.\n(Initialize Stop Notifier)"
        n89 = Unbundle By Name(w272) -> ("SweepControl"=w270:refnum<class "Sweep Control.lvclass">)
        n90 = call <userlib>:"Read Dependencies.vi"("error in (no error)"=w266, "SweepControl in"=w270) -> ("error out"=w265:errorcluster, "Transport"=w268:refnum<class "Transport.lvclass">, "SweepControl out"=w269:refnum<class "Sweep Control.lvclass">)  [unwired: 7 in]
        n91 = call <userlib>:"Init Notifiers.vi"("error in (no error)"=w265, "Transport in"=w268) -> ("error out"=w264:errorcluster, "Transport out"=w267:refnum<class "Transport.lvclass">)  [unwired: 8 in]
        n92 = call <userlib>:"Write Dependencies.vi"("error in (no error)"=w264, "Transport"=w267, "SweepControl in"=w269) -> ("error out"=w263:errorcluster, "SweepControl out"=w271:refnum<class "Sweep Control.lvclass">)  [unwired: 7 in]
        n93 = Bundle By Name(cluster=w272, "SweepControl"=w271) -> (w273:T31)
        n94 = call <vilib>:"Add State(s) to Queue__jki_lib_state_machine.vi"("State(s) in (\"\")"=w275) -> ("States Out"=w274:string)  [unwired: 14 in]
      }
      frame "Sweep: Prepare JSON" {
        # "Sweep: Prepare JSON.\n(Prepare Sweep Configuration data for *.json file)"
        n95 = Unbundle By Name(w300) -> ("SweepControl"=w286:refnum<class "Sweep Control.lvclass">, "B field values"=w284:dbl[], "SweepControl"=w288:refnum<class "Sweep Control.lvclass">, "Instruments.DAQ"=w277:refnum<class "Instrument.LockinAPI.lvclass">, "Instruments.Amplifier"=w280:refnum<class "Instrument.Amplifier.lvclass">)
        n96 = call <userlib>:"Read Dependencies.vi"("error in (no error)"=w283, "SweepControl in"=w288) -> ("error out"=w295:errorcluster, "Transport"=w297:refnum<class "Transport.lvclass">)  [unwired: 7 in, 1 out]
        n97 = call <userlib>:"Read Dependencies.vi"("error in (no error)"=w295, "Transport"=w297) -> ("error out"=w296:errorcluster, "C.E."=w298:refnum<class "Control Experiment.lvclass">)  [unwired: 7 in, 1 out]
        n98 = Unbundle By Name(w286) -> ("Experiment"=w285:T3)
        n99 = To More Specific Class(target class=refnum<class "Instrument.Lockin.lvclass"> refnum ("Instrument.Lockin in"), reference=w277) -> (specific class reference=w276:refnum<class "Instrument.Lockin.lvclass">)  [unwired: 1 in, 1 out]
        n100 = call <userlib>:"Read Experiment Configuration.vi"("error in (no error)"=w296, "Control Experiment in"=w298) -> ("error out"=w304:errorcluster, "Experiment Description"=w293:T13, "Control Experiment out"=w303:refnum<class "Control Experiment.lvclass">)  [unwired: 7 in]
        n101 = To More Specific Class(target class=refnum<class "Inst.Krohn-Hite-7008.lvclass"> refnum ("Inst.Krohn-Hite-7008 in"), reference=w280) -> (specific class reference=w279:refnum<class "Inst.Krohn-Hite-7008.lvclass">)  [unwired: 1 in, 1 out]
        n102 = call <userlib>:"Read Wiring Configuration.vi"("error in (no error)"=w304, "Control Experiment in"=w303) -> ("error out"=w287:errorcluster, "Wiring Configuration"=w289:T16)  [unwired: 7 in, 1 out]
        n103 = call-dynamic "getAOconfig.vi"("error in (no error)"=w283, "Instrument.Lockin in"=w276) -> ("error out"=w305:errorcluster, "AOconfig"=w291:T17, "Instrument.Lockin out"=w306:refnum<class "Instrument.Lockin.lvclass">)  [unwired: 7 in]
        n104 = for {
          N: 1 -> [_]
          tunnel: w279 -> [w312]
          tunnel: [w309] -> w292 mode=concatenating
          tunnel: w283 -> [w310]
          tunnel: [w311] -> w301
          n105 = call-dynamic "Inst.KH7008.getAllChannels.vi"("error in (no error)"=w310, "Inst.Krohn-Hite-7008 in"=w312) -> ("error out"=w311:errorcluster, "allChannelProperties"=w309:T22)  [unwired: 7 in, 1 out]
        }
        n106 = call-dynamic "getREFconfig.vi"("error in (no error)"=w305, "Instrument.Lockin in"=w306) -> ("error out"=w302:errorcluster, "REFconfig"=w290:T20)  [unwired: 7 in, 1 out]
        n107 = Bundle By Name(cluster=w300, "ContinuousB_JSON.Continuous B Sweep.Experiment"=w285, "ContinuousB_JSON.Continuous B Sweep.B field values"=w284, "ContinuousB_JSON.Experiment Description"=w293, "ContinuousB_JSON.Wiring Configuration"=w289, "ContinuousB_JSON.Lockin.AOconfig"=w291, "ContinuousB_JSON.Lockin.REFconfig"=w290, "ContinuousB_JSON.Krohn Hite.Channel Setting"=w292) -> (w299:T31)
        n108 = Merge Errors(w287, w302, w301) -> (w294:errorcluster)
        n109 = call <vilib>:"Add State(s) to Queue__jki_lib_state_machine.vi"("State(s) in (\"\")"=w308) -> ("States Out"=w307:string)  [unwired: 14 in]
      }
      frame "Sweep: Write JSON" {
        # "Sweep: Write JSON.\n(Writes <ContinuousB> json section)"
        n110 = Unbundle By Name(w334) -> ("SweepControl"=w325:refnum<class "Sweep Control.lvclass">, "ContinuousB_JSON"=w317:T12)
        n111 = call <userlib>:"Read Dependencies.vi"("error in (no error)"=w323, "SweepControl in"=w325) -> ("error out"=w322:errorcluster, "Transport"=w332:refnum<class "Transport.lvclass">, "SweepControl out"=w327:refnum<class "Sweep Control.lvclass">)  [unwired: 7 in]
        n112 = call <userlib>:"Read Dependencies.vi"("error in (no error)"=w322, "Transport"=w332) -> ("error out"=w314:errorcluster, "C.E."=w316:refnum<class "Control Experiment.lvclass">, "Transport"=w328:refnum<class "Transport.lvclass">)  [unwired: 7 in]
        n113 = call <userlib>:"Write JSON to Dictionary.vi"("error in (no error)"=w314, "Control Experiment in"=w316) -> ("error out"=w313:errorcluster, "Control Experiment out"=w315:refnum<class "Control Experiment.lvclass">)  [unwired: 8 in]
        n114 = call "To JSON Text.vim"("error in (no error)"=w313, "Anything"=w317) -> ("error out"=w321:errorcluster, "<JSON>"=w331:string)  [unwired: 8 in]
        n115 = call <userlib>:"Write Dictionary Element.vi"("error in (no error)"=w321, "value"=w331, "key"="<ContinuousB>", "Control Experiment in"=w315) -> ("error out"=w320:errorcluster, "Control Experiment out"=w329:refnum<class "Control Experiment.lvclass">)  [unwired: 6 in]
        n116 = call <userlib>:"Write Dependencies.vi"("error in (no error)"=w320, "Control Experiment"=w329, "Transport in"=w328) -> ("error out"=w319:errorcluster, "Transport out"=w326:refnum<class "Transport.lvclass">)  [unwired: 7 in]
        n117 = call <userlib>:"Write Dependencies.vi"("error in (no error)"=w319, "Transport"=w326, "SweepControl in"=w327) -> ("error out"=w318:errorcluster, "SweepControl out"=w324:refnum<class "Sweep Control.lvclass">)  [unwired: 7 in]
        n118 = Bundle By Name(cluster=w334, "SweepControl"=w324) -> (w333:T31)
        n119 = call <vilib>:"Add State(s) to Queue__jki_lib_state_machine.vi"("State(s) in (\"\")"=w336) -> ("States Out"=w335:string)  [unwired: 14 in]
      }
      frame "Sweep: Simulate Sweep" {
        # "Sweep Rate"
        # "B Field Values"
        # "Sweep: Simulate Sweep.\n(Graphical displays B waypoints for user verifaction)"
        n120 = Unbundle By Name(w340) -> ("Sweep rate (T/min)"=w339:dbl, "B field values"=w338:dbl[])
        n121 = Array Size(array=w338) -> (size(s)=w341:i32)
        n122 = Decrement(x=w341) -> (x-1=w342:i32)
        n123 = for {
          N: w342 -> [_]
          tunnel: w339 -> [w364]
          tunnel: w338 -> [w372]
          tunnel: [w365] -> w343 mode=indexing
          i -> [w370]
          n124 = Increment(x=w370) -> (x+1=w371:i32)
          n125 = Index Array(array=w372, index #1=w370, index #2=w371) -> (element #1=w368:dbl, element #2=w369:dbl)
          n126 = Subtract(x=w368, y=w369) -> (x-y=w367:dbl)
          n127 = Absolute Value(x=w367) -> (abs(x)=w366:dbl)
          n128 = Divide(x=w366, y=w364) -> (x/y=w365:dbl)
        }
        n129 = for {
          tunnel: w338 -> [w356] mode=indexing
          i -> [w357]
          stop <- w354 stop-if-true
          n130 = local read "B Field Graph"() -> (w360:cluster{i32[], dbl[]}[])
          n131 = Build Array(w357) -> (w362:i32[])
          n132 = Build Array(w356) -> (w361:dbl[])
          n133 = local read "stop"() -> (w354:bool)
          n134 = Bundle(w362, w361) -> (w358:cluster{i32[], dbl[]})  [unwired: 1 in]
          n135 = local write "Setpoint (T)"(w356) -> ()
          n136 = local write "Step #"(w357) -> ()
          n137 = Index Array(array=w360) -> (element=w359:cluster{i32[], dbl[]})  [unwired: 1 in]
          n138 = Build Array(w359, w358) -> (w355:cluster{i32[], dbl[]}[])
          n139 = local write "B Field Graph"(w355) -> ()
          n140 = call <userlib>:"Wait (ms)__ogtk.vi"("milliseconds to wait"=u32 250) -> ()  [unwired: 9 in, 2 out]
        }
        n141 = Get Date/Time In Seconds() -> (seconds since 1Jan1904=w346:timestamp)
        n142 = Add Array Elements(numeric array=w343) -> (sum=w348:dbl)
        n143 = Quotient & Remainder(x=w348, y=60.0) -> (x-y*floor(x/y)=→"time (minutes)":dbl, floor(x/y)=→"time (hours)":dbl)
        n144 = Multiply(x=w348, y=60.0) -> (x*y=w345:dbl)
        n145 = Add(x=w345, y=w346) -> (x+y=→"ETA":timestamp)
        n146 = call <vilib>:"Add State(s) to Queue__jki_lib_state_machine.vi"("State(s) in (\"\")"=w353) -> ("States Out"=w352:string)  [unwired: 14 in]
      }
      frame "Sweep: Execute" {
        # "Sweep: Execute.\n(Start sweep B from start to finish while continuously taking measurements)"
        n147 = Unbundle By Name(w380) -> ("Instruments.Magnet"=w387:refnum<class "Instrument.Cryostat.lvclass">, "B field values"=w376:dbl[], "Sweep rate (T/min)"=w388:dbl, "Transport"=w389:refnum<class "Transport.lvclass">, "SweepControl"=w377:refnum<class "Sweep Control.lvclass">)
        n148 = Bundle By Name(cluster=w377, "Lockin_Sweep Configuration"="Lockin_sweep Configuration") -> (w385:refnum<class "Sweep Control.lvclass">)
        n149 = while {
          tunnel: w389 -> [w404]
          tunnel: w386 -> [w417]
          tunnel: [w401] -> w384
          shift-right: [w424] -> _
          shift-left: 0 -> [w421]
          tunnel: w376 -> [w411]
          tunnel: w388 -> [w409]
          tunnel: "Mode" -> [w413]
          shift-right: [w412] -> w378
          shift-left: w387 -> [w416]
          tunnel: [w403] -> w375
          i -> [w420]
          stop <- w405 stop-if-true
          # "setpoint"
          # "ramp rate"
          # "Loop that sends notifications"
          n150 = Array Size(array=w411) -> (size(s)=w419:i32)
          n151 = Decrement(x=w419) -> (x-1=w422:i32)
          n152 = Index Array(array=w411, index=w421) -> (element=w410:dbl)
          "Setpoint (T)" <- w410
          n153 = Greater Or Equal?(x=w420, y=w422) -> (x >= y?=w423:bool)
          n154 = Or(x="stop", y=w423) -> (x .or. y?=w425:bool)
          n155 = Or(x=w425, y=w417) -> (x .or. y?=w405:bool)
          n156 = call-dynamic "setMagnet.vi"("Mode"=w413, "Axis"=Magnet_Axis--Enum."Z", "error in (no error)"=w417, "Target Rate (T/min)"=w409, "Target Field (T)"=w410, "Instrument.Cryostat in"=w416) -> ("error out"=w414:errorcluster, "Instrument.Cryostat out"=w415:refnum<class "Instrument.Cryostat.lvclass">)  [unwired: 4 in]
          n157 = call-dynamic "waitForMagnet.vi"("Axis"=Magnet_Axis--Enum."Z", "error in (no error)"=w414, "Tolerance (T)"=0.001, "Setpoint (T)"=w410, "Instrument.Cryostat in"=w415) -> ("error out"=w402:errorcluster, "Instrument.Cryostat out"=w412:refnum<class "Instrument.Cryostat.lvclass">)  [unwired: 5 in]
          n158 = call <userlib>:"Send Stop Notifier.vi"("error in (no error)"=w402, "Stop [T]"=w405, "Transport in"=w404) -> ("error out"=w401:errorcluster, "Transport out"=w403:refnum<class "Transport.lvclass">)  [unwired: 7 in]
          n159 = Increment(x=w421) -> (x+1=w424:i32)
          "Step #" <- w420
        }
        n160 = while {
          tunnel: w386 -> [w398]
          tunnel: w389 -> [w396]
          tunnel: [w399] -> w383
          tunnel: w385 -> [w397]
          stop <- w400 stop-if-true
          # "Loop that listens to notifications"
          n161 = call "Take Measurement.vi"("error in (no error)"=w398, "SweepControl in"=w397) -> ("error out"=w393:errorcluster)  [unwired: 8 in, 1 out]
          n162 = call <userlib>:"Get Stop Notifier.vi"("error in (no error)"=w393, "Transport in"=w396) -> ("error out"=w394:errorcluster, "Stop?"=w395:bool)  [unwired: 7 in, 1 out]
          n163 = Or(x=w395, y=w394) -> (x .or. y?=w400:bool)
          n164 = call <vilib>:"Clear Errors.vi"("error in (no error)"=w394) -> ("error out"=w399:errorcluster)  [unwired: 5 in, 1 out]
        }
        n165 = Bundle By Name(cluster=w380, "Instruments.Magnet"=w378) -> (w379:T31)
        n166 = Merge Errors(w384, w383) -> (w374:errorcluster)
        n167 = call <userlib>:"Destroy Notifiers.vi"("error in (no error)"=w374, "Transport in"=w375) -> ("error out"=w373:errorcluster)  [unwired: 9 in]
        n168 = call <vilib>:"Add State(s) to Queue__jki_lib_state_machine.vi"("State(s) in (\"\")"=w392) -> ("States Out"=w391:string)  [unwired: 14 in]
      }
    }
  }
  "error out" <- w1
